vi "Camera Found.vi"(8 "error in":errorcluster, 11 "CameraName":string) -> (0 "error out":errorcluster, 2 "Camera Found":bool, 3 "CameraName out":string)   [LabVIEW 2012]
uses:
  <vilib>/vision/driver/NI_Vision_Acquisition_Software.lvlib
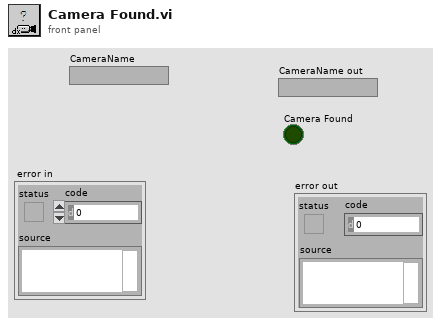
[diagram p1: front panel]
types:
  T1 = cluster{"Type":u32, "Version":u32, "Flags":u32, "SerialNumberHigh":u32, "SerialNumberLow":u32, "BusType":u32, "InterfaceName":string, "VendorName":string, "ModelName":string, "CameraFileName":string, "CameraAttributeURL":string}[]
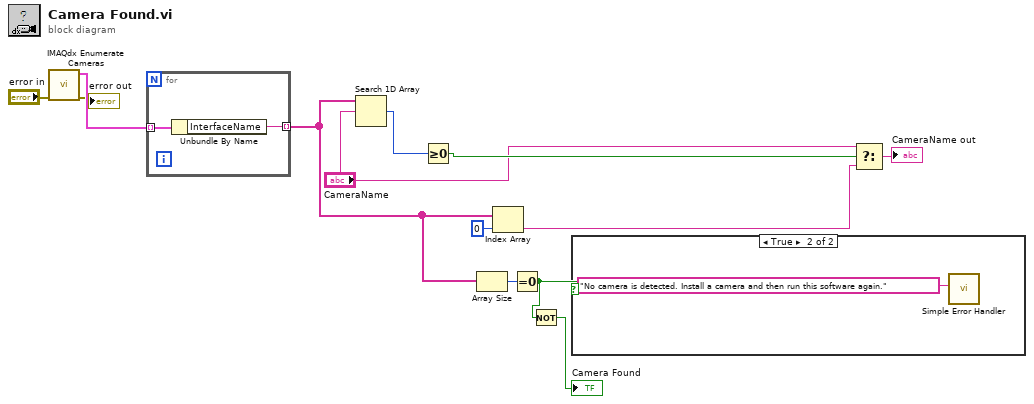
[diagram p0: block diagram]
diagram:
  n1 = call <vilib>:"IMAQdx Enumerate Cameras.vi"("error in"="error in") -> ("error out"=→"error out":errorcluster, "Camera Information Array"=w13:T1)  [unwired: 9 in]
  n2 = for {
    tunnel: w13 -> [w15] mode=indexing
    tunnel: [w14] -> w4 mode=indexing
    n3 = Unbundle By Name(w15) -> ("InterfaceName"=w14:string)
  }
  n4 = Search 1D Array(1D array=w4, element="CameraName") -> (index of element=w12:i32)  [unwired: 1 in]
  n5 = Greater Or Equal To 0?(x=w12) -> (x >= 0?=w10:bool)
  n6 = Array Size(array=w4) -> (size(s)=w3:i32)
  n7 = Index Array(array=w4, index=0) -> (element=w8:string)
  n8 = Equal To 0?(x=w3) -> (x = 0?=w2:bool)
  n9 = Not(x=w2) -> (.not. x?=→"Camera Found":bool)
  n10 = case shown="True" w2 {
    frame False {
    }
    frame True {
      n11 = call <vilib>:"Simple Error Handler.vi"("error source (\" \")"="No camera is detected. Install a camera and then run this software again." ("error source (\" \")")) -> ()  [unwired: 4 in, 5 out]
    }
  }
  n12 = Select(t="CameraName", s=w10, f=w8) -> (s? t:f=→"CameraName out":string)
